vi "CANopenReadSDO.vi"(0 "FPGA VI Reference In":refnum<k20>, 1 "ID":u32=1408, 2 "error in":errorcluster) -> (3 "FPGA VI Reference Out":refnum<k20>, 4 "Timestamp":dbl, 5 "Data":u8[](array[numeric]), 6 "error out":errorcluster)   [LabVIEW 2016]
doc: "This VI serves as a SUB VI for the Read+ VI."
uses:
  <vilib>/Utility/error.llb/Error Cluster From Error Code.vi
  <vilib>/rvi/errors/niLvFpgaAdjustHostInterfaceError.vi
  <vilib>/rvi/interface/nirviReadWriteControl/nirviReadWriteControl.xnode
  FPGA Bitfiles/EV-MCU_FPGATarget_CANEngine(FPGA)b_eM8Xz3qYJVA.lvbitx
  CAN_Engine(FPGA)_basic.vi
  NiFpgaLv.dll
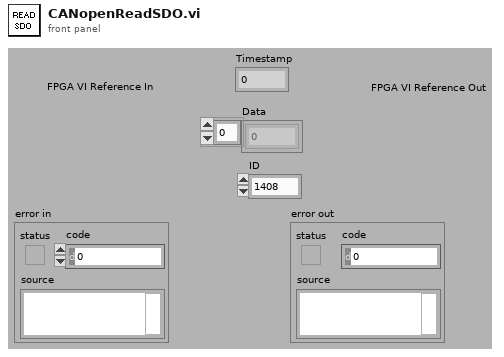
[diagram p1: front panel]
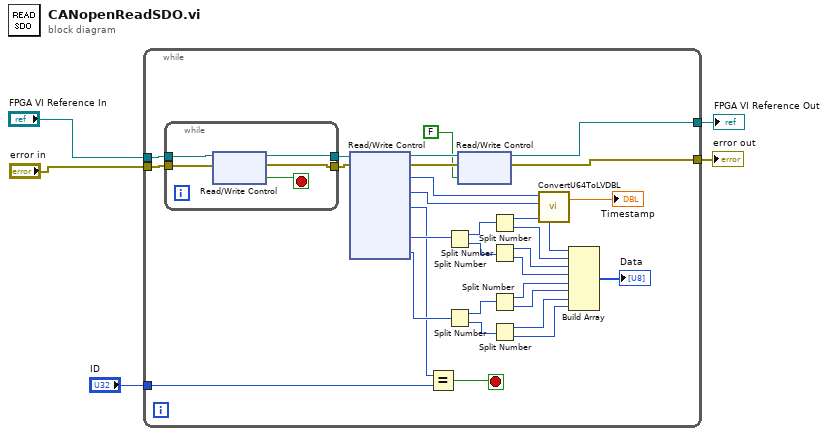
[diagram p0: block diagram]
diagram:
  n1 = while {
    tunnel: "FPGA VI Reference In" -> [w15]
    tunnel: "error in" -> [w14]
    tunnel: [w11] -> w3
    tunnel: [w10] -> w2
    tunnel: "ID" -> [w6]
    stop <- w7 stop-if-true
    n2 = while {
      tunnel: w14 -> [w38]
      tunnel: w15 -> [w39]
      tunnel: [w40] -> w35
      tunnel: [w37] -> w34
      stop <- w36 stop-if-true
      n3 = xnode "Read/Write Control"("FPGA VI Reference In"=w39, "error in"=w38) -> ("FPGA VI Reference Out"=w40:refnum<k20>, "error out"=w37:errorcluster, "Ready"=w36:bool)
    }
    n4 = xnode "Read/Write Control"("FPGA VI Reference In"=w35, "error in"=w34) -> ("FPGA VI Reference Out"=w13:refnum<k20>, "error out"=w12:errorcluster, "U32 In"=w21:u32, "U32 In 2"=w20:u32, "U32 In 3"=w8:u32, "U32 In 5"=w18:u32, "U32 In 6"=w17:u32)  [unwired: 1 out]
    n5 = Equal?(x=w8, y=w6) -> (x = y?=w7:bool)
    n6 = Split Number(x=w18) -> (hi(x)=w22:u16, lo(x)=w23:u16)
    n7 = Split Number(x=w17) -> (hi(x)=w25:u16, lo(x)=w24:u16)
    n8 = xnode "Read/Write Control"("FPGA VI Reference In"=w13, "error in"=w12, "Ready"=FALSE) -> ("FPGA VI Reference Out"=w11:refnum<k20>, "error out"=w10:errorcluster)
    n9 = Split Number(x=w22) -> (hi(x)=w26:u8, lo(x)=w27:u8)
    n10 = Split Number(x=w23) -> (hi(x)=w28:u8, lo(x)=w29:u8)
    n11 = Split Number(x=w25) -> (hi(x)=w30:u8, lo(x)=w31:u8)
    n12 = Split Number(x=w24) -> (hi(x)=w32:u8, lo(x)=w33:u8)
    n13 = call "ConvertU64ToLVDBL.vi"("Time U64 LowPart"=w20, "Time U64 HighPart"=w21) -> ("Time LV DBL"=→"Timestamp":dbl)  [unwired: 3 in]
    n14 = Build Array(w26, w27, w28, w29, w30, w31, w32, w33) -> (→"Data":u8[])
  }
  "error out" <- w2
  "FPGA VI Reference Out" <- w3
